vi "String shared Variable Test.vi"(6 "Value":string, 8 "error in (no error)":errorcluster, 9 "shared variable refnum":refnum<k21>="ni.var.psp://localhost/Test Shared Variables/Bool") -> (0 "error out":errorcluster)   [LabVIEW 2021]
uses:
  Source/STR/conc_SharedVar_STR.lvclass
  <vilib>/TSA/Abstract Data Classes/Abs_Types/String/Abs_String.lvclass
  C:/Program Files (x86)/National Instruments/LabVIEW 2021/vi.lib/TSA/Abstract Data Classes/Abs_Types/Type/Abs_Type.lvclass
  <vilib>/TSA/Abstract Data Classes/Abs_Types/String/Static Read.vi
  <vilib>/TSA/Abstract Data Classes/Abs_Types/String/Static Write.vi
  9c5f5204-69d5-44b0-9fed-84ac97b71057.vi
  103af6e5-0f20-4bd9-87ce-4bacf20ebd2f.vi
  <vilib>/addons/_JKI Toolkits/Caraya/classes/Assert/Assert Equal Value_Variant.vi
  <vilib>/addons/_JKI Toolkits/Caraya/classes/Assert/Assert Equal Type_Variant.vi
  <vilib>/TSA/Abstract Data Classes/Abs_Types/Type/Abs_Type.lvclass
  <vilib>/addons/_JKI Toolkits/Caraya/classes/Test/Test.lvclass
  <vilib>/Utility/Data Type/NI_Data Type.lvlib
  <vilib>/addons/_JKI Toolkits/Caraya/classes/Assert/Assert.lvclass
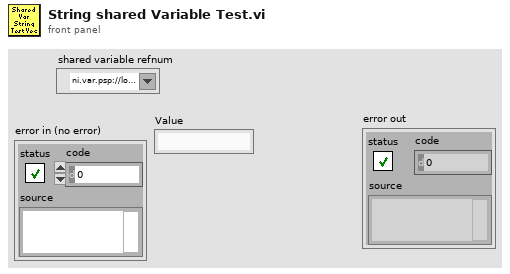
[diagram p1: front panel]
types:
  T1 = typedef "NI_Data Type.lvlib/Data Type.ctl" = enum8{"Invalid Type", "Void", "I8", "I16", "I32", "I64", "U8", "U16", "U32", "U64", "Single Float", "Double Float", "Extended Float", "Single Complex", "Double Complex", "Extended Complex", "Enum U8", "Enum U16", "Enum U32", "Enum U64", "Single Float With Unit", "Double Float With Unit", "Extended Float With Unit", "Single Complex with Unit", "Double Complex with Unit", "Extended Complex with Unit", "Boolean", "String", "Path", "Picture", "Tag", "Array", "Cluster", "Variant", "LV Variant", "Waveform", "Timestamp", "Digital Waveform", "Digital Data", "ExpressData", "Refnum", "External Data", "VI", "Poly VI", "LabVIEW Class Instance", "Fixed Point", "Set Collection", "Map Collection"}
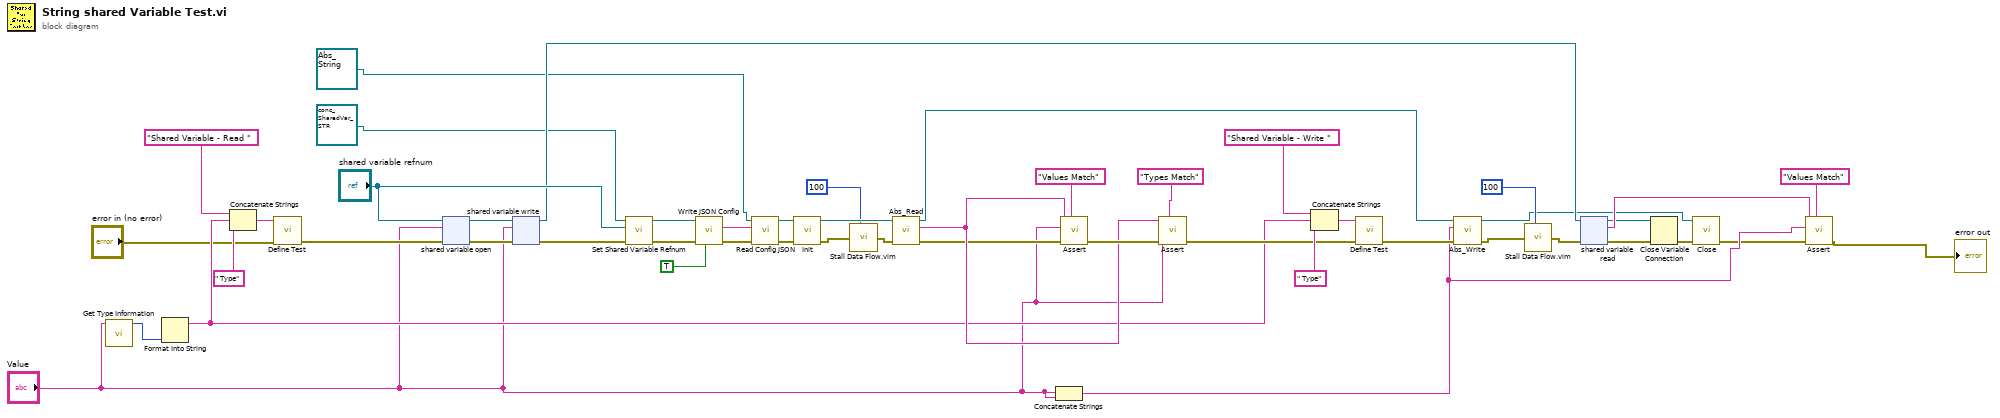
[diagram p0: block diagram]
diagram:
  n1 = call <vilib>:"Get Type Information.vi"("variant"="Value") -> ("type"=w38:T1)  [unwired: 6 in, 4 out]
  n2 = Format Into String(w38) -> (resulting string=w24:string)  [unwired: 3 in, 1 out]
  n3 = Concatenate Strings("Shared Variable - Read " ("string"), w24, " Type" ("string")) -> (w37:string)
  n4 = call <vilib>:"Define Test.vi"("error in (no error)"="error in (no error)", "Label (VI Title)"=w37) -> ("error out"=w29:errorcluster)  [unwired: 8 in, 1 out]
  n5 = shared-variable-open("shared variable refnum", w29, "Value") -> (w49:refnum<k21>, w48:errorcluster)  [unwired: 1 in]
  n6 = shared-variable-write(w49, w48, "Value") -> (w17:refnum<k21>, w47:errorcluster)
  n7 = call-dynamic "Set Shared Variable Refnum.vi"("error in (no error)"=w47, "shared variable refnum"="shared variable refnum", "abs_SharedVar_Bool in"=refnum<class "conc_SharedVar_STR.lvclass"> refnum ("conc_SharedVar_STR.lvclass")) -> ("error out"=w44:errorcluster, "abs_SharedVar_Bool out"=w45:refnum<class "conc_SharedVar_STR.lvclass">)  [unwired: 7 in]
  n8 = call-dynamic "Write JSON Config.vi"("Pretty Print?"=TRUE, "error in (no error)"=w44, "abs_SharedVar_Bool in"=w45) -> ("error out"=w39:errorcluster, "JSON"=w40:string)  [unwired: 6 in, 1 out]
  n9 = call <vilib>:"Read Config JSON.vi"("error in (no error)"=w39, "JSON Config"=w40, "Abs_Type in"=refnum<class "Abs_String.lvclass"> refnum ("Abs_String.lvclass")) -> ("error out"=w42:errorcluster, "Abs_Type out"=w41:refnum<class "Abs_String.lvclass">)  [unwired: 7 in]
  n10 = call-dynamic "Init.vi"("error in (no error)"=w42, "Data in"=w41) -> ("error out"=w12:errorcluster, "Data out"=w31:refnum<class "Abs_String.lvclass">)  [unwired: 8 in]
  n11 = call "Stall Data Flow.vim"("value in"=w12, "milliseconds to wait"=u32 100) -> ("value out"=w11:errorcluster)  [unwired: 1 out]
  n12 = call-poly <vilib>:"Abs_Read.vi"("error in (no error)"=w11, "Abs_String in"=w31) -> ("error out"=w28:errorcluster, "String"=w30:string, "Abs_String out"=w21:refnum<class "Abs_String.lvclass">)  [unwired: 7 in]
  n13 = Concatenate Strings("Value", "Value") -> (w14:string)
  n14 = call-poly <vilib>:"Assert.vi"("Label"="Values Match", "error in (no error)"=w28, "Y"="Value", "X"=w30) -> ("error out"=w34:errorcluster)  [unwired: 6 in, 1 out]
  n15 = call-poly <vilib>:"Assert.vi"("Label"="Types Match", "error in (no error)"=w34, "Y"="Value", "X"=w30) -> ("error out"=w25:errorcluster)  [unwired: 6 in, 1 out]
  n16 = Concatenate Strings("Shared Variable - Write " ("string"), w24, " Type" ("string")) -> (w26:string)
  n17 = call <vilib>:"Define Test.vi"("error in (no error)"=w25, "Label (VI Title)"=w26) -> ("error out"=w22:errorcluster)  [unwired: 8 in, 1 out]
  n18 = call-poly <vilib>:"Abs_Write.vi"("error in (no error)"=w22, "String"=w14, "Abs_String in"=w21) -> ("error out"=w20:errorcluster, "Abs_String out"=w5:refnum<class "Abs_String.lvclass">)  [unwired: 7 in]
  n19 = call "Stall Data Flow.vim"("value in"=w20, "milliseconds to wait"=u32 100) -> ("value out"=w19:errorcluster)  [unwired: 1 out]
  n20 = shared-variable-read(w17, w19) -> (w7:refnum<k21>, w8:errorcluster, w15:string)  [unwired: 1 out]
  n21 = Close Variable Connection(8:w8, 11:w7) -> (0:w6:errorcluster)
  n22 = call-dynamic "Close.vi"("error in (no error)"=w6, "Data in"=w5) -> ("error out"=w1:errorcluster)  [unwired: 8 in, 1 out]
  n23 = call-poly <vilib>:"Assert.vi"("Label"="Values Match", "error in (no error)"=w1, "Y"=w14, "X"=w15) -> ("error out"=→"error out":errorcluster)  [unwired: 6 in, 1 out]
